vi "Store Double Curves.vi"(2 "N":i32=1, 3 "No. of Run":i32, 4 "Element in":dbl, 5 "Array in":dbl[](array[numeric]), 6 "Action":T2=enum."Set", 7 "Curve Index":T1 items=["Frequency (GHz)", "THz Photo Current (nA)"]) -> (0 "data set no. (= row index)":i32, 1 "Array out":dbl[](array[numeric]))   [LabVIEW 2013]
uses:
  Store Data Actions.ctl
  Variables.ctl
panel:
  in  "No. Rows":i32=1000
  in  "No. Columns":i32=12
  in  "No. Runs":i32=1
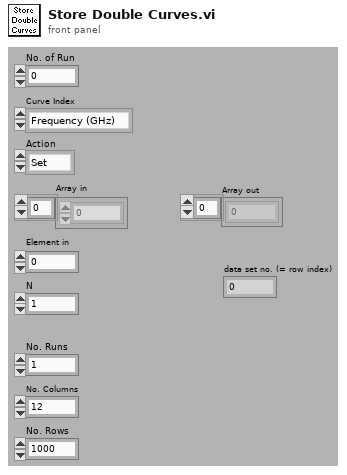
[diagram p1: front panel]
types:
  T1 = typedef "Variables.ctl" = i32
  T2 = typedef "Store Data Actions.ctl" = enum16{"Init", "Set", "Add", "Add Array", "Read", "Row+N"}
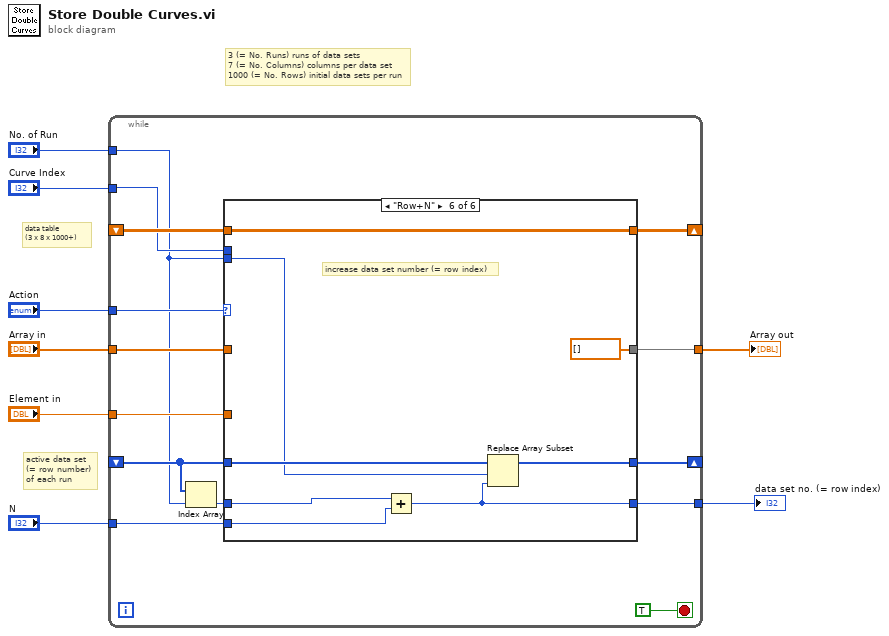
[diagram p0: block diagram]
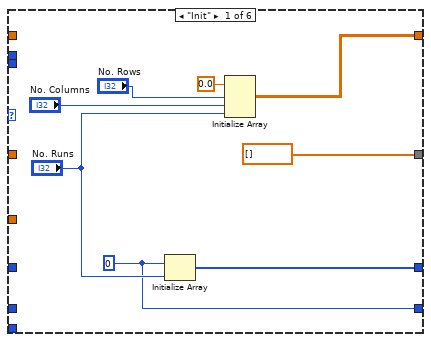
[diagram p2: hidden frame]
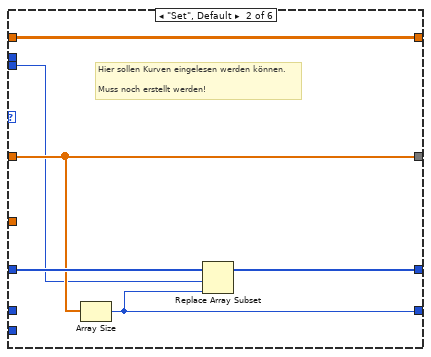
[diagram p3: hidden frame]
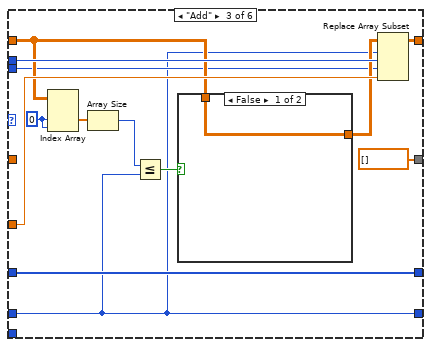
[diagram p4: hidden frame]
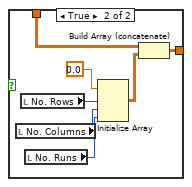
[diagram p5: hidden frame]
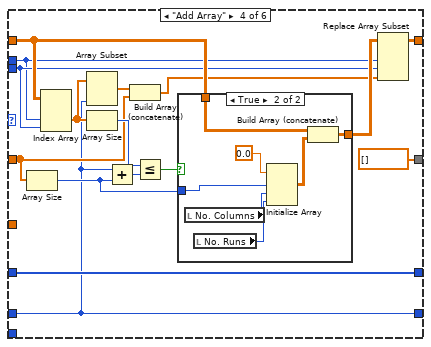
[diagram p6: hidden frame]
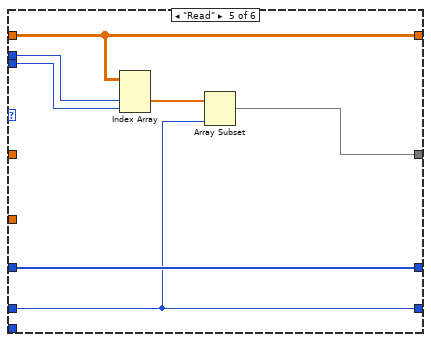
[diagram p8: hidden frame]
diagram:
  # "data table\n(3 x 8 x 1000+)"
  # "active data set\n(= row number)\nof each run"
  # "3 (= No. Runs) runs of data sets\n7 (= No. Columns) columns per data set\n1000 (= No. Rows) initial data sets per run"
  n1 = while {
    shift-right: [w15] -> _
    shift-left: _ -> [w18]
    tunnel: "Action" -> [w21]
    tunnel: "Array in" -> [w20]
    tunnel: "Curve Index" -> [w14]
    tunnel: [w17] -> w4
    tunnel: "Element in" -> [w19]
    tunnel: "No. of Run" -> [w11]
    shift-right: [w16] -> _
    shift-left: _ -> [w12]
    tunnel: [w13] -> w2
    tunnel: "N" -> [w9]
    stop <- TRUE stop-if-true
    n2 = Index Array(array=w12, index=w11) -> (element=w10:i32)
    n3 = case shown="\"Row+N\"" w21 {
      tunnel: [dbl[] [] ("f") w34 dbl[] [] dbl[] [] w84 dbl[] []] -> w17
      tunnel: w20 -> [_ w34 _ w61 _ _]
      tunnel: w19 -> [_ _ w48 _ _ _]
      tunnel: [w29 w36 w49 w73 w88 w96] -> w15
      tunnel: w18 -> [_ w36 w42 w68 w88 w96]
      tunnel: [w28 w33 w46 w72 w85 w94] -> w16
      tunnel: w12 -> [_ w35 w46 w72 w85 w93]
      tunnel: w11 -> [_ w31 w39 w66 w83 w91]
      tunnel: w14 -> [_ _ w47 w65 w87 _]
      tunnel: [w23 w32 w37 w58 w82 w92] -> w13
      tunnel: w10 -> [_ _ w37 w58 w82 w90]
      tunnel: w9 -> [_ _ _ _ _ w89]
      frame "Init" {
        w23 = 0
        n4 = Initialize Array(w23, "No. Runs") -> (w28:i32[])
        n5 = Initialize Array(0.0, "No. Rows", "No. Columns", "No. Runs") -> (w29:dbl[][][])
      }
      frame "Set", Default {
        # "Hier sollen Kurven eingelesen werden können.\n\nMuss noch erstellt werden!"
        n6 = Array Size(array=w34) -> (size(s)=w32:i32)
        n7 = Replace Array Subset(array=w35, new element=w32, index=w31) -> (w33:i32[])
      }
      frame "Add" {
        w38 = 0 ("index (page)")
        n8 = Index Array(array=w42, index (dim 1)=w38, index (dim 2)=w38) -> (element=w41:dbl[])  [unwired: 1 in]
        n9 = Array Size(array=w41) -> (size(s)=w40:i32)
        n10 = Less Or Equal?(x=w40, y=w37) -> (x <= y?=w44:bool)
        n11 = case shown="False" w44 {
          tunnel: w42 -> [w50 w56]
          tunnel: [w50 w57] -> w43
          frame False {
          }
          frame True {
            n12 = local read "No. Columns"() -> (w53:i32)
            n13 = local read "No. Rows"() -> (w51:i32)
            n14 = local read "No. Runs"() -> (w52:i32)
            n15 = Initialize Array(0.0 ("element"), w51, w53, w52) -> (w55:dbl[][][])
            n16 = Build Array (concatenate)(w56, w55) -> (w57:dbl[][][])
          }
        }
        n17 = Replace Array Subset(array=w43, new element=w48, index (dim 0)=w37, index (dim 1)=w47, index (dim 2)=w39) -> (w49:dbl[][][])
      }
      frame "Add Array" {
        n18 = Array Size(array=w61) -> (size(s)=w59:i32)
        n19 = Index Array(array=w68, index (dim 1)=w65, index (dim 2)=w66) -> (element=w64:dbl[])  [unwired: 1 in]
        n20 = Array Subset(array=w64, length=w58) -> (w62:dbl[])  [unwired: 1 in]
        n21 = Array Size(array=w64) -> (size(s)=w67:i32)
        n22 = Add(x=w58, y=w59) -> (x+y=w63:i32)
        n23 = Build Array (concatenate)(w62, w61) -> (w60:dbl[])
        n24 = Less Or Equal?(x=w67, y=w63) -> (x <= y?=w70:bool)
        n25 = case shown="True" w70 {
          tunnel: w68 -> [w74 w80]
          tunnel: [w74 w81] -> w69
          tunnel: w59 -> [_ w75]
          frame False {
          }
          frame True {
            n26 = local read "No. Columns"() -> (w77:i32)
            n27 = local read "No. Runs"() -> (w76:i32)
            n28 = Initialize Array(0.0 ("element"), w75, w77, w76) -> (w79:dbl[][][])
            n29 = Build Array (concatenate)(w80, w79) -> (w81:dbl[][][])
          }
        }
        n30 = Replace Array Subset(array=w69, new element=w60, index (dim 1)=w65, index (dim 2)=w66) -> (w73:dbl[][][])  [unwired: 1 in]
      }
      frame "Read" {
        n31 = Index Array(array=w88, index (dim 1)=w87, index (dim 2)=w83) -> (element=w86:dbl[])  [unwired: 1 in]
        n32 = Array Subset(array=w86, length=w82) -> (w84:dbl[])  [unwired: 1 in]
      }
      frame "Row+N" {
        # "increase data set number (= row index)"
        n33 = Add(x=w90, y=w89) -> (x+y=w92:i32)
        n34 = Replace Array Subset(array=w93, new element=w92, index=w91) -> (w94:i32[])
      }
    }
  }
  "Array out" <- w4
  "data set no. (= row index)" <- w2
